vi "WFRepetitionsAssemble.vi"(9 "Repeat":i32=1, 10 "Interval (s)":dbl min=0.0, 11 "Delay (s)":dbl min=0.0) -> (3 "Repetitions":T1={"Delay (s)"=0.0, "Interval (s)"=0.0, "Repeat"=1} {"Interval (s)" min=0.0; "Delay (s)" min=0.0})   [LabVIEW 2009]
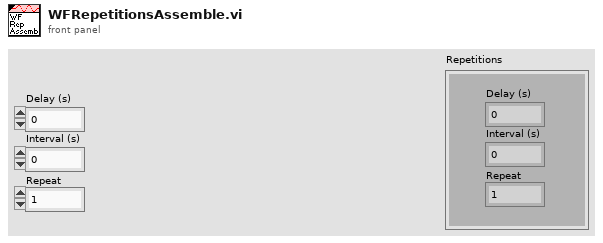
[diagram p1: front panel]
types:
  T1 = cluster{"Delay (s)":dbl, "Interval (s)":dbl, "Repeat":i32}
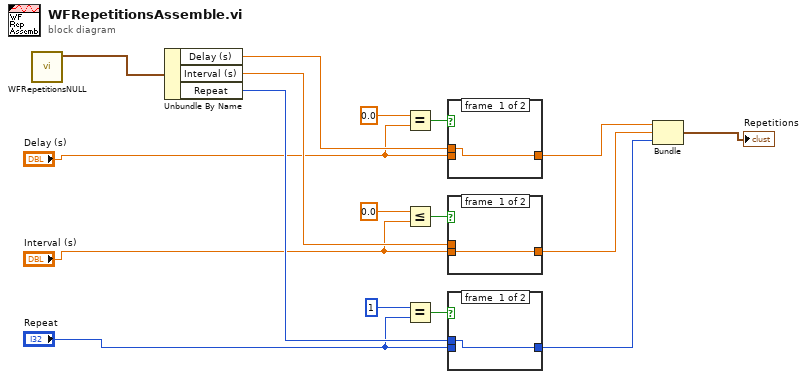
[diagram p0: block diagram]
diagram:
  n1 = call "WFRepetitionsNULL.vi"() -> ("Repetitions"=w5:T1)  [unwired: 11 in]
  n2 = Unbundle By Name(w5) -> ("Delay (s)"=w7:dbl, "Interval (s)"=w11:dbl, "Repeat"=w14:i32)
  n3 = Equal?(x=0.0, y="Delay (s)") -> (x = y?=w9:bool)
  n4 = Less Or Equal?(x=0.0, y="Interval (s)") -> (x <= y?=w13:bool)
  n5 = Equal?(x=1, y="Repeat") -> (x = y?=w17:bool)
  n6 = case shown="False" w9 {
    tunnel: "Delay (s)" -> [_ w19]
    tunnel: [w18 w19] -> w6
    tunnel: w7 -> [w18 _]
    frame #0 {
    }
    frame #1 {
    }
  }
  n7 = case shown="False" w13 {
    tunnel: "Interval (s)" -> [w20 _]
    tunnel: [w20 w21] -> w10
    tunnel: w11 -> [_ w21]
    frame #0 {
    }
    frame #1 {
    }
  }
  n8 = case shown="True" w17 {
    tunnel: "Repeat" -> [_ w23]
    tunnel: [w22 w23] -> w15
    tunnel: w14 -> [w22 _]
    frame #0 {
    }
    frame #1 {
    }
  }
  n9 = Bundle("Delay (s)"=w6, "Interval (s)"=w10, "Repeat"=w15) -> (→"Repetitions":T1)  [unwired: 1 in]
